vi "GetClassAndFunc.vi"(8 "error in (no error)":errorcluster caption="entrée d'erreur", 11 "ClassType":enum16{"BaseDevices", "Instruments"}(ring)) -> (0 "error out":errorcluster, 1 "ClassFuncCtrl":path[](array[path]), 2 "ClassNames":string[](array[string]), 3 "AllFunctions":string[](array[string]), 4 "FuncNamesArr":string[][](array[string]))   [LabVIEW 2019]
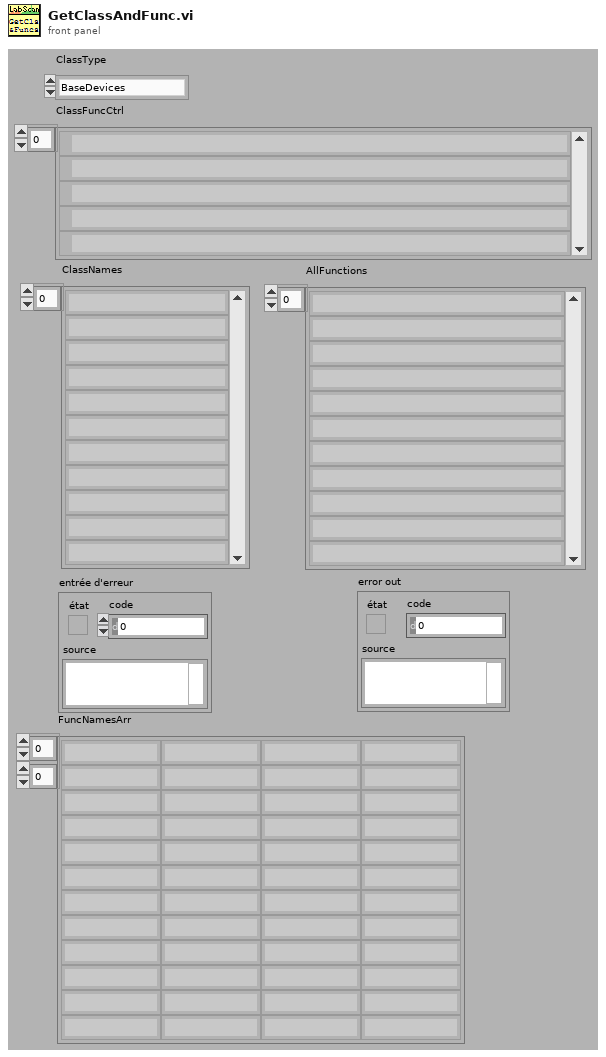
[diagram p1: front panel]
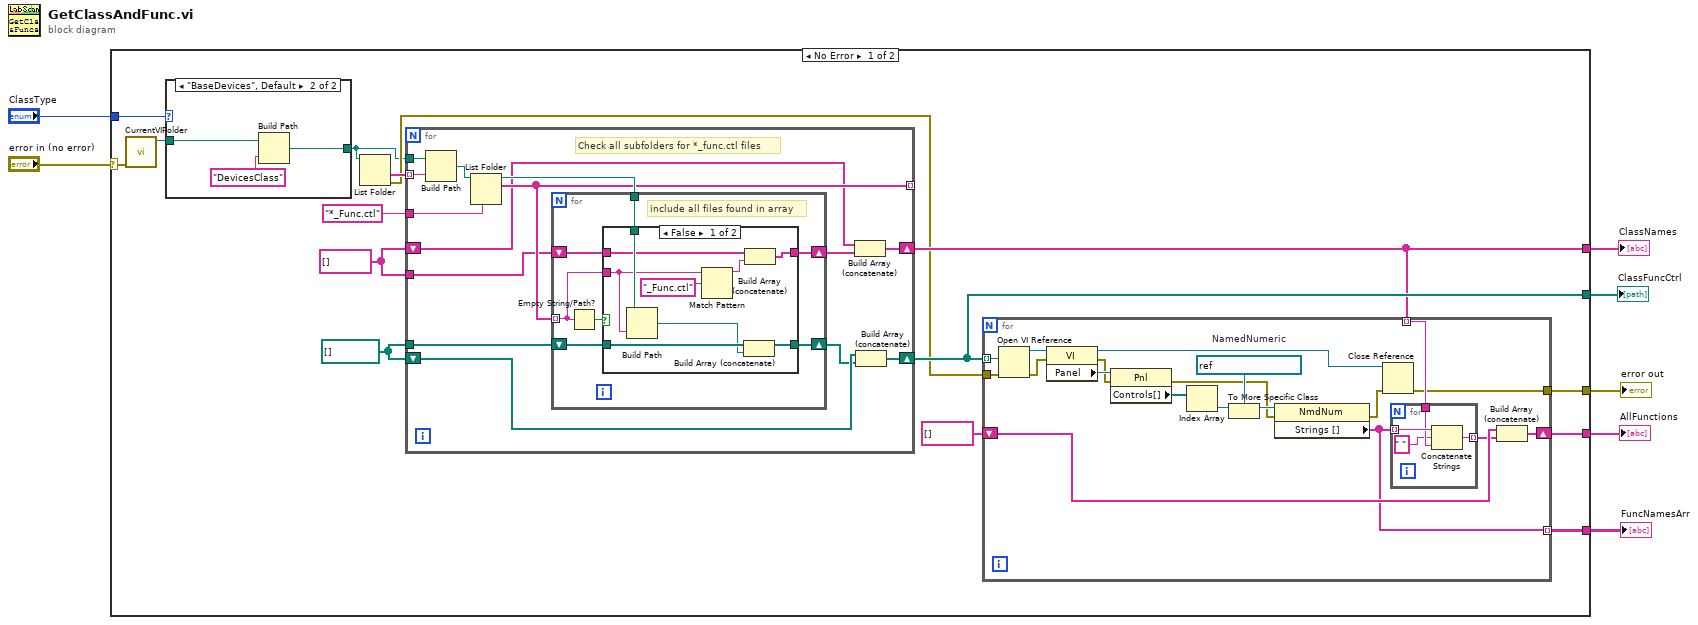
[diagram p0: block diagram]
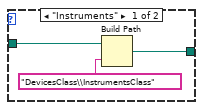
[diagram p2: hidden frame]
diagram:
  n1 = case shown="No Error" "error in (no error)" {
    selector: "error in (no error)" -> [w12 w84]
    tunnel: [w20 _] -> w7
    tunnel: [w19 _] -> w6
    tunnel: [w16 _] -> w5
    tunnel: [w14 w84] -> w4
    tunnel: [w11 _] -> w2
    tunnel: "ClassType" -> [w9 _]
    frame No Error {
      w17 = string[] []
      w15 = path[] []
      n2 = call <userlib>:"CurrentVIFolder.vi"("error in (no error)"=w12) -> ("Chemin"=w10:path)  [unwired: 8 in, 2 out]
      n3 = case shown="\"BaseDevices\", Default" w9 {
        tunnel: w10 -> [w25 w28]
        tunnel: [w24 w26] -> w8
        frame "Instruments" {
          n4 = Build Path(base path=w25, name or relative path="DevicesClass\\InstrumentsClass" ("nom ou chemin relatif")) -> (appended path=w24:path)
        }
        frame "BaseDevices", Default {
          n5 = Build Path(base path=w28, name or relative path="DevicesClass" ("nom ou chemin relatif")) -> (appended path=w26:path)
        }
      }
      n6 = List Folder(path=w8) -> (folder names=w22:string[], error out=w13:errorcluster)  [unwired: 3 in, 2 out]
      n7 = for {
        tunnel: w22 -> [w64] mode=indexing
        tunnel: w8 -> [w65]
        tunnel: "*_Func.ctl" ("filtre") -> [w52]
        tunnel: [w61] -> _ mode=indexing
        shift-right: [w53] -> w20
        shift-left: w15 -> [w59]
        tunnel: w15 -> [w60]
        shift-right: [w56] -> w19
        shift-left: w17 -> [w55]
        tunnel: w17 -> [w54]
        # "Check all subfolders for *_func.ctl files"
        n8 = Build Path(base path=w65, name or relative path=w64) -> (appended path=w63:path)
        n9 = List Folder(path=w63, pattern=w52) -> (path out=w62:path, filenames=w61:string[])  [unwired: 2 in, 2 out]
        n10 = for {
          tunnel: w62 -> [w72]
          tunnel: w61 -> [w69] mode=indexing
          shift-right: [w71] -> w58
          shift-left: w60 -> [w68]
          shift-right: [w67] -> w57
          shift-left: w54 -> [w66]
          # "include all files found in array"
          n11 = Empty String/Path?(string/path=w69) -> (empty?=w70:bool)
          n12 = case shown="False" w70 {
            tunnel: w72 -> [w81 _]
            tunnel: w69 -> [w75 _]
            tunnel: [w80 w83] -> w71
            tunnel: w68 -> [w79 w83]
            tunnel: [w77 w82] -> w67
            tunnel: w66 -> [w76 w82]
            frame False {
              n13 = Build Path(base path=w81, name or relative path=w75) -> (appended path=w78:path)
              n14 = Match Pattern(string=w75, regular expression="_Func.ctl" ("expression régulière")) -> (before substring=w73:string)  [unwired: 1 in, 3 out]
              n15 = Build Array (concatenate)(w79, w78) -> (w80:path[])
              n16 = Build Array (concatenate)(w76, w73) -> (w77:string[])
            }
            frame True {
            }
          }
        }
        n17 = Build Array (concatenate)(w55, w57) -> (w56:string[])
        n18 = Build Array (concatenate)(w59, w58) -> (w53:path[])
      }
      n19 = for {
        tunnel: w20 -> [w47] mode=indexing
        tunnel: w19 -> [w34] mode=indexing
        shift-right: [w38] -> w16
        shift-left: string[] [] ("Strings []") -> [w39]
        tunnel: w13 -> [w31]
        tunnel: [w30] -> w14
        tunnel: [w29] -> w11 mode=indexing
        w42 = refnum<vi> refnum  # NamedNumeric
        n20 = Open VI Reference(vi path=w47, error in (no error)=w31) -> (vi reference=w46:refnum<vi>, error out=w36:errorcluster)  [unwired: 4 in]
        n21 = property class="VI"(reference=w46, error in=w36) -> (reference out=w44:refnum<vi>, error out=w35:errorcluster, "Panel"=w45:refnum<vi>)
        n22 = property class="Pnl"(reference=w45, error in=w35) -> (error out=w33:errorcluster, "Controls[]"=w41:refnum<vi>[])  [unwired: 1 out]
        n23 = Index Array(array=w41) -> (element=w40:refnum<vi>)  [unwired: 1 in]
        n24 = To More Specific Class(target class=w42, reference=w40) -> (specific class reference=w43:refnum<vi>)  [unwired: 1 in, 1 out]
        n25 = property class="NmdNum"(reference=w43, error in=w33) -> (error out=w32:errorcluster, "Strings []"=w29:string[])  [unwired: 1 out]
        n26 = Close Reference(reference=w44, error in (no error)=w32) -> (error out=w30:errorcluster)
        n27 = for {
          tunnel: w29 -> [w51] mode=indexing
          tunnel: w34 -> [w50]
          tunnel: [w49] -> w37 mode=indexing
          n28 = Concatenate Strings(w51, " " ("chaîne"), w50) -> (w49:string)
        }
        n29 = Build Array (concatenate)(w39, w37) -> (w38:string[])
      }
    }
    frame Error {
    }
  }
  "ClassNames" <- w6
  "ClassFuncCtrl" <- w7
  "AllFunctions" <- w5
  "error out" <- w4
  "FuncNamesArr" <- w2
